vi "Fetch PRACH EVM Vs Preamble Trace Results.vi"(8 "error in (no error)":errorcluster, 10 "Instance (1)":T1=1, 11 "VISA resource name":refnum<visa-resource-name>) -> (0 "error out":errorcluster, 1 "Results":dbl[](array[numeric]) format="%^.3e", 2 "Reliability":i32, 3 "VISA resource name out":refnum<visa-resource-name>)   [LabVIEW 2020, in "Rohde&Schwarz CMWXP NR FR1 Measurement.lvlib"]
doc: "Returns the values of the EVM vs preamble traces.\n\nAttribute:\nRSCMWXPNRFR1M_ATTR_FETCH_PRACH_EVM_VS_PREAMBLE_TRACE_RESULTS\n\nRemote-control command:\nFETCh:NRSub:MEAS<i>:PRACh:TRACe:EVPReamble?"
uses:
  <instrlib>/Rohde&Schwarz CMWXP NR FR1 Measurement/Rohde&Schwarz CMWXP NR FR1 Measurement.lvlib
  <instrlib>/Rohde&Schwarz CMWXP NR FR1 Measurement/Private/_Instance.ctl
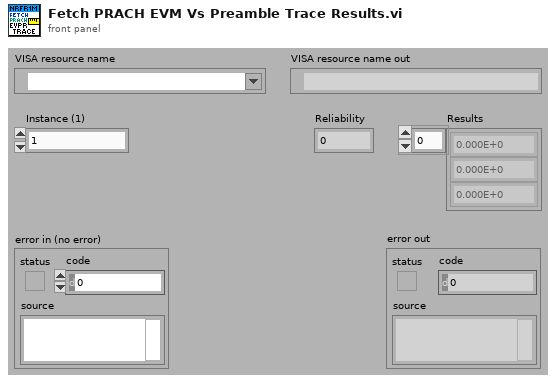
[diagram p1: front panel]
types:
  T1 = typedef "Rohde&Schwarz CMWXP NR FR1 Measurement.lvlib/_Instance.ctl" = i32
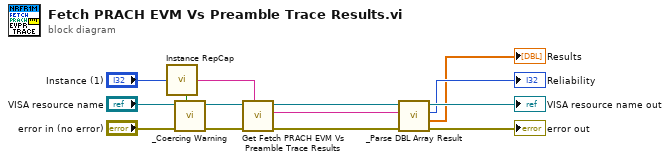
[diagram p0: block diagram]
diagram:
  n1 = call <instrlib>:"Instance RepCap.vi"("Instance In"="Instance (1)") -> ("In Range?"=w14:bool, "RepCap Identifier Out"=w8:string)  [unwired: 1 in]
  n2 = call <instrlib>:"_Coercing Warning.vi"("In Range?"=w14, "error in (no error)"="error in (no error)", "VISA resource name"="VISA resource name") -> ("error out"=w11:errorcluster, "VISA resource name out"=w10:refnum<visa-resource-name>)  [unwired: 7 in]
  n3 = call "Get Fetch PRACH EVM Vs Preamble Trace Results"("Repeated Capabilities"=w8, "error in (no error)"=w11, "instrument handle"=w10) -> ("error out"=w7:errorcluster, "Fetch PRACH EVM Vs Preamble Trace Results"=w3:string, "instrument handle out"=w4:refnum<visa-resource-name>)  [unwired: 6 in]
  n4 = call <instrlib>:"_Parse DBL Array Result.vi"("error in (no error)"=w7, "Input String"=w3, "VISA resource name"=w4) -> ("error out"=→"error out":errorcluster, "Results"=→"Results":dbl[], "Reliability"=→"Reliability":i32, "VISA resource name out"=→"VISA resource name out":refnum<visa-resource-name>)  [unwired: 5 in]
